vi "ControlPanel.vi"(0 "NXT":T1={"Hardware"="NXT", "Flattened String"=""}) -> (5 "NXT":T1={"Hardware"="NXT", "Flattened String"=""})   [LabVIEW 2010]
uses:
  <vilib>/NXT/Block Support/NXT_InputPort.ctl
  <vilib>/NXT/Subs/LVHSConnector.ctl
  <vilib>/NXT/Block Support/NXT_ButtonSelector.ctl
  <vilib>/NXT/Subs/MotorXNode.DC Motor Type.ctl
  <vilib>/NXT/NXTIO Xnodes/NXTIOXNode/NXTIO.xnode
  <vilib>/NXT/Subs/MotorXNode.1DCMotor.ctl
  <vilib>/NXT/Subs/MotorXNode.Servo Type.ctl
  <vilib>/NXT/Subs/MotorXNode.1Servo.ctl
  <vilib>/NXT/Dual Mode Library/Waits/Wait_Num(msec).vi
  <vilib>/NXT/Dual Mode Library/Display/clearDisplay.vi
  <vilib>/NXT/Dual Mode Library/Waits/Wait_Btn_Release.vi
  <vilib>/NXT/Dual Mode Library/Display/drawText.vi
  <vilib>/NXT/Dual Mode Library/Display/drawNumber.vi
  <vilib>/NXT/Dual Mode Library/Display/drawNumber_float.vi
  <vilib>/NXT/NXTIO Xnodes/NXTIONodeSubVIs/TETRIX IO Move DC Motors.vi
  <vilib>/NXT/NXTIO Xnodes/NXTIONodeSubVIs/TETRIX IO Motor Status.vi
  <vilib>/NXT/NXTIO Xnodes/NXTIONodeSubVIs/TETRIX IO Move Servos.vi
  Components/Components.lvlib
panel:
  out "exit?":bool
  out "Enter":bool caption="Yes/No"
  out "Right":bool caption="Yes/No"
  out "Left":bool caption="Yes/No"
  in  "Sensor Type":T2(ring)
  in  "MUX Port":u8(ring) items=["No MUX", "MUX 1", "MUX 2", "MUX 3", "MUX 4"]
  in  "Sensor Port":T3 items=["Port 1", "Port 2", "Port 3", "Port 4"]
  in  "Motor Port":u8(ring)=1 items=["A", "B", "C"]
  in  "Type":T4(ring)
  in  "Controller Slot":u8(ring)=1 items=["1"=1, "2"=2, "3"=3, "4"=4, "5"=5, "6"=6]
  in  "Chain Position":u8(ring)=1 items=["1"=1, "2"=2, "3"=3, "4"=4]
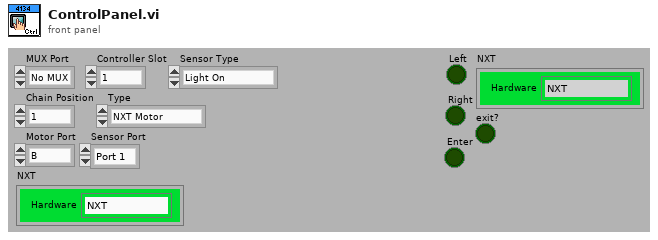
[diagram p1: front panel]
types:
  T1 = typedef "LVHSConnector.ctl" = cluster{"Hardware":string, "Flattened String":string}
  T2 = enum16{"Light On", "Light Off", "Touch", "Sound", "Ultrasonic", "Accelerometer", "Compass", "EOPD", "Force", "Gyro", "IR v1", "IR v2"}
  T3 = typedef "NXT_InputPort.ctl" = u8
  T4 = enum16{"NXT Motor", "NXT Rotation Sensor", "NXT Sensor", "NXT Battery", "Tetrix Motor", "Tetrix Servo", "Tetrix Encoder", "Tetrix Battery"}
  T5 = typedef "MotorXNode.DC Motor Type.ctl" = enum16{"DC Motor"}
  T6 = typedef "MotorXNode.Servo Type.ctl" = enum16{"Servo"}
  T7 = cluster{"Direction (0-9)":i16, "Signal Strength (Array)":u8[]}
  T8 = typedef "NXT_ButtonSelector.ctl" = u16
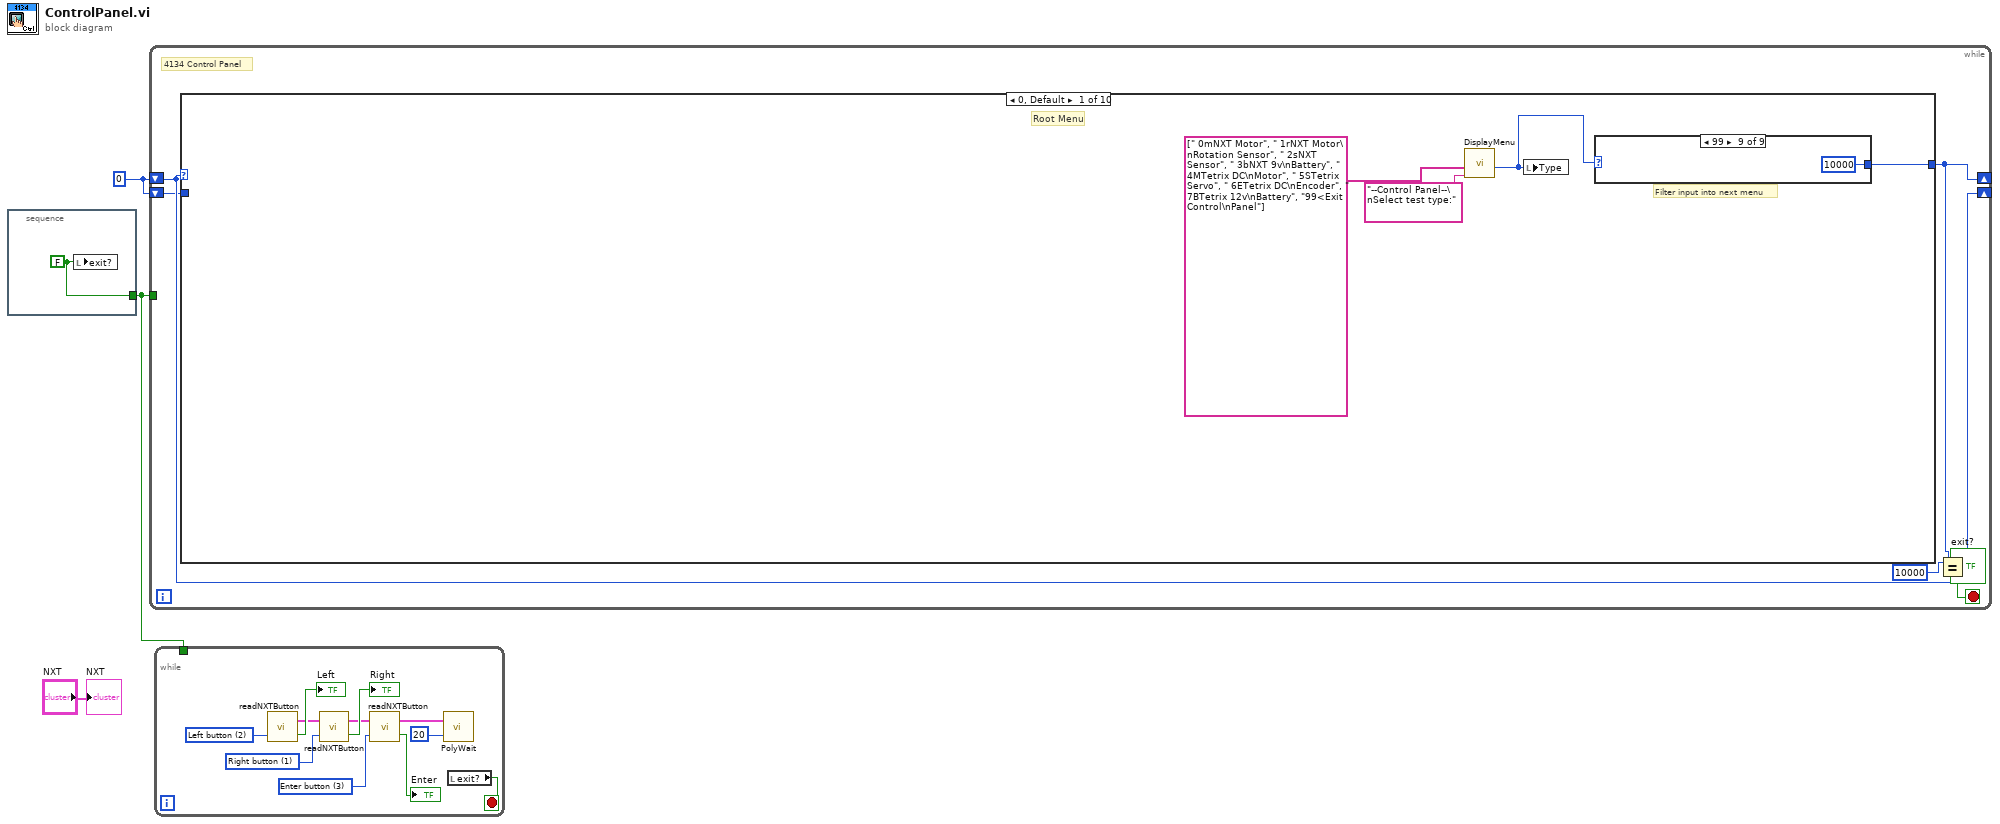
[diagram p0: block diagram]
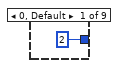
[diagram p2: hidden frame]
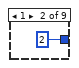
[diagram p3: hidden frame]
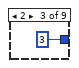
[diagram p4: hidden frame]
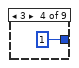
[diagram p5: hidden frame]
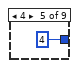
[diagram p6: hidden frame]
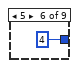
[diagram p7: hidden frame]
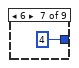
[diagram p8: hidden frame]
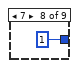
[diagram p9: hidden frame]
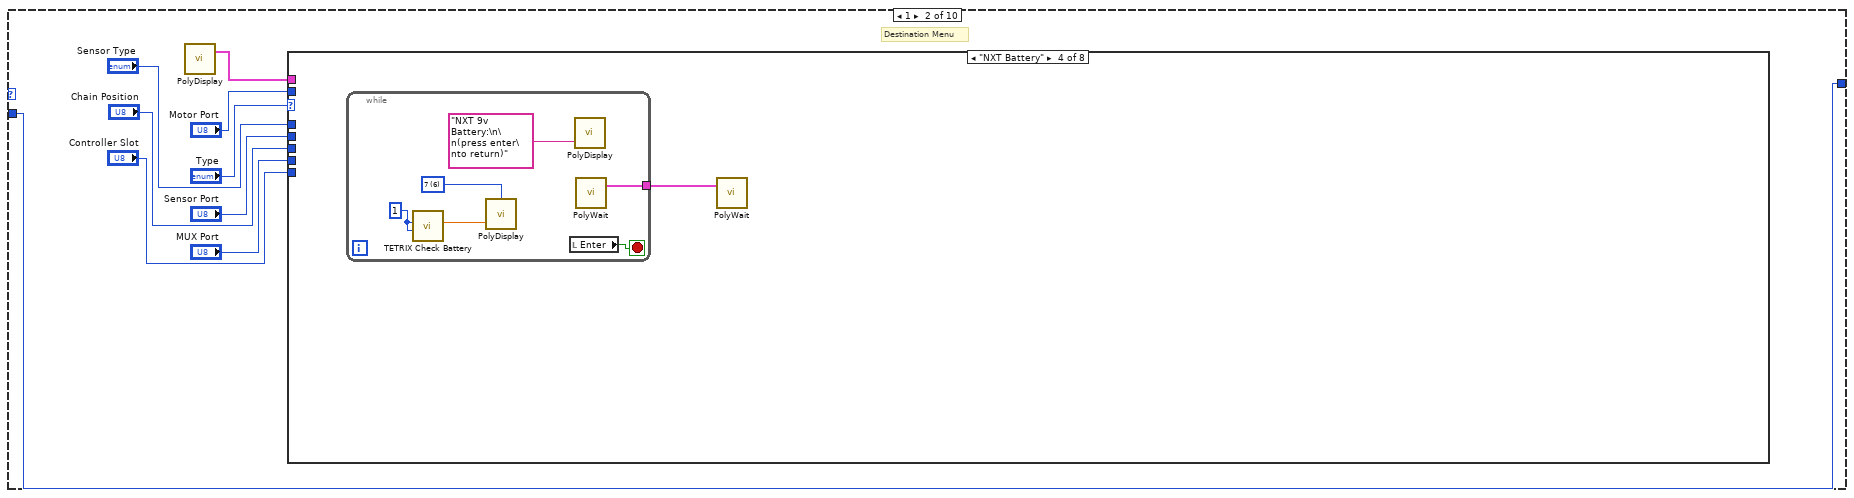
[diagram p10: hidden frame]
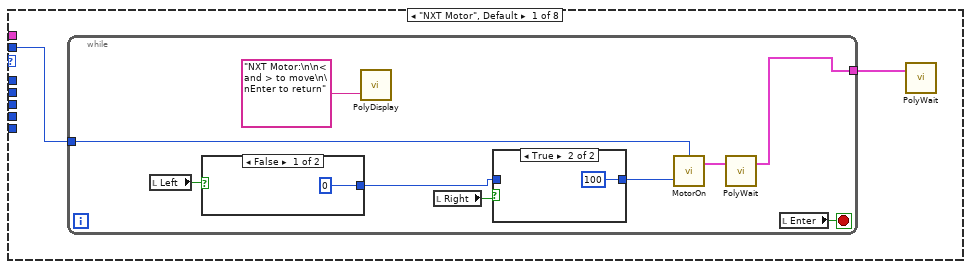
[diagram p11: hidden frame]
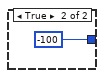
[diagram p13: hidden frame]
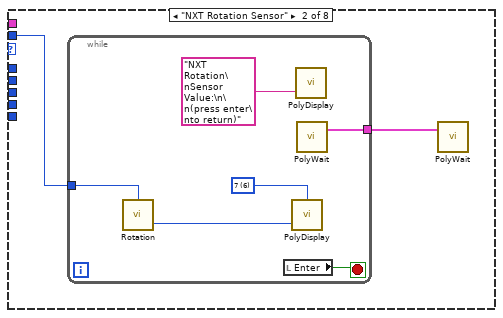
[diagram p14: hidden frame]
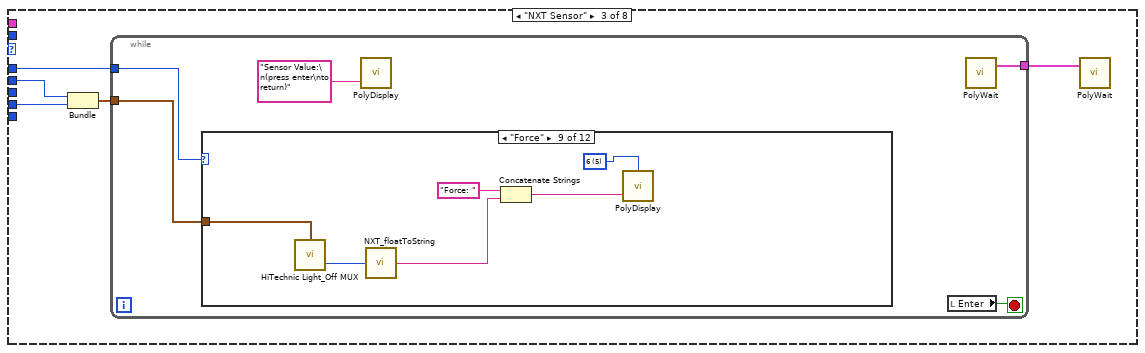
[diagram p15: hidden frame]
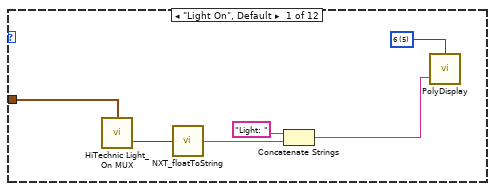
[diagram p16: hidden frame]
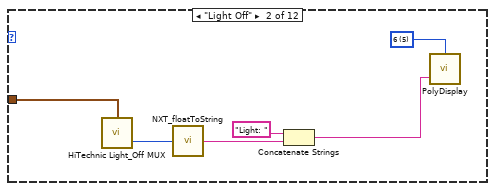
[diagram p17: hidden frame]
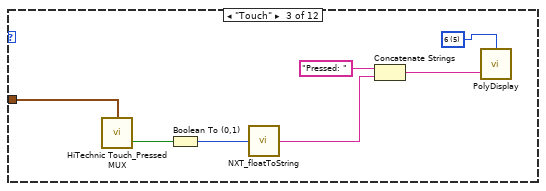
[diagram p18: hidden frame]
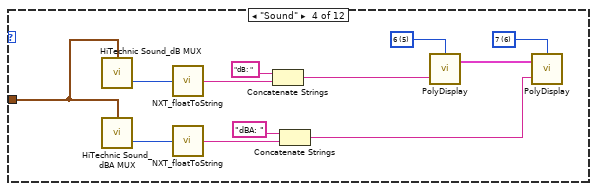
[diagram p19: hidden frame]
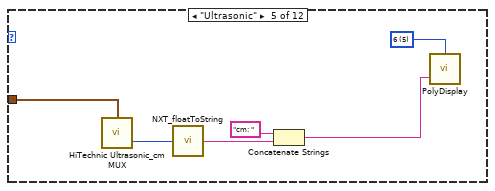
[diagram p20: hidden frame]
diagram:
  w3 = u32 0 ("Selected ID")
  n1 = stacked-sequence {
    tunnel: [w4] -> w1
    frame #0 {
      w4 = FALSE ("exit?")
      n2 = local write "exit?"(w4) -> ()
    }
  }
  n3 = while {
    shift-right: [w7] -> _
    shift-left: w3 -> [w9]
    shift-right: [w9] -> _
    shift-left: w3 -> [w8]
    tunnel: w1 -> [_]
    stop <- w6 stop-if-true
    # "4134 Control Panel"
    n4 = case shown="0, Default" w9 {
      tunnel: [w11 w30 w336 w343 w350 w357 w366 w375 w382 w389] -> w7
      tunnel: w8 -> [_ w30 _ _ _ _ _ _ _ _]
      frame 0, Default {
        # "Filter input into next menu"
        # "Root Menu"
        n5 = call "DisplayMenu.vi"("Menu Message"="--Control Panel--\nSelect test type:", "2-Digit ID+Character+Message"=string[] [" 0mNXT Motor", " 1rNXT Motor\nRotation Sensor", " 2sNXT Sensor", " 3bNXT 9v\nBattery", " 4MTetrix DC\nMotor", " 5STetrix Servo", " 6ETetrix DC\nEncoder", " 7BTetrix 12v\nBattery", "99<Exit Control\nPanel"] ("Array")) -> ("Selected ID"=w12:i32)  [unwired: 6 in, 1 out]
        n6 = local write "Type"(w12) -> ()
        n7 = case shown="99" w12 {
          tunnel: [2 2 3 1 4 4 4 1 10000] -> w11
          frame 0, Default {
          }
          frame 1 {
          }
          frame 2 {
          }
          frame 3 {
          }
          frame 4 {
          }
          frame 5 {
          }
          frame 6 {
          }
          frame 7 {
          }
          frame 99 {
          }
        }
      }
      frame 1 {
        # "Destination Menu"
        n8 = call-poly <vilib>:"PolyDisplay.vi"() -> ("NXT"=w29:T1)  [unwired: 4 in]
        n9 = case shown="\"NXT Battery\"" "Type" {
          tunnel: w29 -> [_ _ _ _ _ _ _ _]
          tunnel: "Motor Port" -> [w32 w47 _ _ _ _ _ _]
          tunnel: "Sensor Port" -> [_ _ w57 _ w188 w223 w269 _]
          tunnel: "MUX Port" -> [_ _ w58 _ _ _ _ _]
          tunnel: "Chain Position" -> [_ _ _ _ w185 w220 w266 _]
          tunnel: "Controller Slot" -> [_ _ _ _ w184 w219 w265 _]
          tunnel: "Sensor Type" -> [_ _ w59 _ _ _ _ _]
          frame "NXT Motor", Default {
            n10 = while {
              tunnel: [w41] -> w33
              tunnel: w32 -> [w38]
              stop <- w34 stop-if-true
              n11 = local read "Left"() -> (w36:bool)
              n12 = case shown="False" w36 {
                tunnel: [0 -100] -> w40
                frame False {
                }
                frame True {
                }
              }
              n13 = call-poly <vilib>:"PolyDisplay.vi"("Text"="NXT Motor:\n\n< and > to move\n\nEnter to return") -> ()  [unwired: 3 in, 1 out]
              n14 = local read "Right"() -> (w35:bool)
              n15 = case shown="True" w35 {
                tunnel: w40 -> [w43 _]
                tunnel: [w43 100] -> w39
                frame False {
                }
                frame True {
                }
              }
              n16 = call <vilib>:"MotorOn.vi"("Power (75)"=w39, "Output Port (All Ports)"=w38) -> ("NXT"=w37:T1)  [unwired: 2 in]
              n17 = call-poly <vilib>:"PolyWait.vi"("NXT"=w37) -> ("NXT"=w41:T1)  [unwired: 3 in]
              n18 = local read "Enter"() -> (w34:bool)
            }
            n19 = call-poly <vilib>:"PolyWait.vi"("NXT"=w33) -> ()  [unwired: 3 in, 1 out]
          }
          frame "NXT Rotation Sensor" {
            n20 = while {
              tunnel: [w52] -> w48
              tunnel: w47 -> [w50]
              stop <- w49 stop-if-true
              w54 = i16 6 items=["1", "2", "3", "4", "5", "6", "7", "8"] ("Line")
              n21 = call <vilib>:"Rotation.vi"("Port (Port A)"=w50) -> ("Angle of Rotation"=w51:i32)  [unwired: 2 in, 1 out]
              n22 = local read "Enter"() -> (w49:bool)
              n23 = call-poly <vilib>:"PolyDisplay.vi"("number"=w51, "Line"=w54) -> ()  [unwired: 2 in, 1 out]
              n24 = call-poly <vilib>:"PolyDisplay.vi"("Text"="NXT Rotation\nSensor Value:\n\n(press enter\nto return)") -> ()  [unwired: 3 in, 1 out]
              n25 = call-poly <vilib>:"PolyWait.vi"() -> ("NXT"=w52:T1)  [unwired: 4 in]
            }
            n26 = call-poly <vilib>:"PolyWait.vi"("NXT"=w48) -> ()  [unwired: 3 in, 1 out]
          }
          frame "NXT Sensor" {
            n27 = Bundle("Sensor Port"=w57, "MUX Port"=w58) -> (w56:cluster{"Sensor Port":T3, "MUX Port":u8})  [unwired: 1 in]
            n28 = while {
              tunnel: w59 -> [w62]
              tunnel: w56 -> [w61]
              tunnel: [w64] -> w55
              stop <- w60 stop-if-true
              n29 = case shown="\"Force\"" w62 {
                tunnel: w61 -> [w70 w71 w79 w90 w96 w118 w120 w129 w138 w144 w152 w161]
                frame "Light On", Default {
                  w65 = i16 5 items=["1", "2", "3", "4", "5", "6", "7", "8"] ("Line")
                  n30 = call <vilib>:"HiTechnic Light_On MUX.vi"("Port/MUX"=w70) -> ("Scaled Value"=w69:i16)  [unwired: 2 in, 1 out]
                  n31 = call <vilib>:"NXT_floatToString.vi"("number"=w69) -> ("string"=w68:string)
                  n32 = Concatenate Strings("Light: ", w68) -> (w66:string)
                  n33 = call-poly <vilib>:"PolyDisplay.vi"("Text"=w66, "Line"=w65) -> ()  [unwired: 2 in, 1 out]
                }
                frame "Light Off" {
                  w72 = i16 5 items=["1", "2", "3", "4", "5", "6", "7", "8"] ("Line")
                  n34 = call <vilib>:"HiTechnic Light_Off MUX.vi"("Port/MUX"=w71) -> ("Scaled Value"=w76:i16)  [unwired: 2 in, 1 out]
                  n35 = call <vilib>:"NXT_floatToString.vi"("number"=w76) -> ("string"=w75:string)
                  n36 = Concatenate Strings("Light: ", w75) -> (w73:string)
                  n37 = call-poly <vilib>:"PolyDisplay.vi"("Text"=w73, "Line"=w72) -> ()  [unwired: 2 in, 1 out]
                }
                frame "Touch" {
                  w80 = i16 5 items=["1", "2", "3", "4", "5", "6", "7", "8"] ("Line")
                  n38 = call <vilib>:"HiTechnic Touch_Pressed MUX.vi"("Port/MUX"=w79) -> ("Yes / No"=w78:bool)  [unwired: 2 in, 1 out]
                  n39 = Boolean To (0,1)(Boolean=w78) -> (0, 1=w77:i16)
                  n40 = call <vilib>:"NXT_floatToString.vi"("number"=w77) -> ("string"=w83:string)
                  n41 = Concatenate Strings("Pressed: ", w83) -> (w81:string)
                  n42 = call-poly <vilib>:"PolyDisplay.vi"("Text"=w81, "Line"=w80) -> ()  [unwired: 2 in, 1 out]
                }
                frame "Sound" {
                  w84 = i16 6 items=["1", "2", "3", "4", "5", "6", "7", "8"] ("Line")
                  w91 = i16 5 items=["1", "2", "3", "4", "5", "6", "7", "8"] ("Line")
                  n43 = call <vilib>:"HiTechnic Sound_dB MUX.vi"("Port/MUX"=w90) -> ("Scaled Value"=w95:i16)  [unwired: 2 in, 1 out]
                  n44 = call <vilib>:"HiTechnic Sound_dBA MUX.vi"("Port/MUX"=w90) -> ("Scaled Value"=w89:i16)  [unwired: 2 in, 1 out]
                  n45 = call <vilib>:"NXT_floatToString.vi"("number"=w95) -> ("string"=w94:string)
                  n46 = call <vilib>:"NXT_floatToString.vi"("number"=w89) -> ("string"=w88:string)
                  n47 = Concatenate Strings("dB: ", w94) -> (w92:string)
                  n48 = Concatenate Strings("dBA: ", w88) -> (w85:string)
                  n49 = call-poly <vilib>:"PolyDisplay.vi"("Text"=w92, "Line"=w91) -> ("NXT"=w86:T1)  [unwired: 2 in]
                  n50 = call-poly <vilib>:"PolyDisplay.vi"("Text"=w85, "NXT"=w86, "Line"=w84) -> ()  [unwired: 1 in, 1 out]
                }
                frame "Ultrasonic" {
                  w97 = i16 5 items=["1", "2", "3", "4", "5", "6", "7", "8"] ("Line")
                  n51 = call <vilib>:"HiTechnic Ultrasonic_cm MUX.vi"("Port/MUX"=w96) -> ("Distance (cm)"=w101:i16)  [unwired: 2 in, 1 out]
                  n52 = call <vilib>:"NXT_floatToString.vi"("number"=w101) -> ("string"=w100:string)
                  n53 = Concatenate Strings("cm: ", w100) -> (w98:string)
                  n54 = call-poly <vilib>:"PolyDisplay.vi"("Text"=w98, "Line"=w97) -> ()  [unwired: 2 in, 1 out]
                }
                frame "Accelerometer" {
                  w114 = i16 7 items=["1", "2", "3", "4", "5", "6", "7", "8"] ("Line")
                  w115 = i16 6 items=["1", "2", "3", "4", "5", "6", "7", "8"] ("Line")
                  w119 = i16 5 items=["1", "2", "3", "4", "5", "6", "7", "8"] ("Line")
                  n55 = call <vilib>:"HiTechnic Acceleration Sensor.vi"("Port/MUX"=w118) -> ("Z Acceleration (m/s^2)"=w102:sgl, "Y Acceleration (m/s^2)"=w105:sgl, "X Acceleration (m/s^2)"=w107:sgl)  [unwired: 3 in, 1 out]
                  n56 = call <vilib>:"NXT_floatToString.vi"("number"=w107) -> ("string"=w106:string)
                  n57 = call <vilib>:"NXT_floatToString.vi"("number"=w105) -> ("string"=w104:string)
                  n58 = call <vilib>:"NXT_floatToString.vi"("number"=w102) -> ("string"=w103:string)
                  n59 = Concatenate Strings("X: ", w106) -> (w111:string)
                  n60 = Concatenate Strings("Y: ", w104) -> (w113:string)
                  n61 = Concatenate Strings("Z: ", w103) -> (w112:string)
                  n62 = call-poly <vilib>:"PolyDisplay.vi"("Text"=w111, "Line"=w119) -> ("NXT"=w117:T1)  [unwired: 2 in]
                  n63 = call-poly <vilib>:"PolyDisplay.vi"("Text"=w113, "NXT"=w117, "Line"=w115) -> ("NXT"=w116:T1)  [unwired: 1 in]
                  n64 = call-poly <vilib>:"PolyDisplay.vi"("Text"=w112, "NXT"=w116, "Line"=w114) -> ()  [unwired: 1 in, 1 out]
                }
                frame "Compass" {
                  w121 = i16 5 items=["1", "2", "3", "4", "5", "6", "7", "8"] ("Line")
                  n65 = call <vilib>:"HiTechnic Compass Sensor.vi"("Port/MUX"=w120) -> ("Heading (degrees)"=w125:i16)  [unwired: 2 in, 1 out]
                  n66 = call <vilib>:"NXT_floatToString.vi"("number"=w125) -> ("string"=w124:string)
                  n67 = Concatenate Strings("Deg: ", w124) -> (w122:string)
                  n68 = call-poly <vilib>:"PolyDisplay.vi"("Text"=w122, "Line"=w121) -> ()  [unwired: 2 in, 1 out]
                }
                frame "EOPD" {
                  w126 = i16 6 items=["1", "2", "3", "4", "5", "6", "7", "8"] ("Line")
                  w133 = i16 5 items=["1", "2", "3", "4", "5", "6", "7", "8"] ("Line")
                  n69 = call <vilib>:"HiTechnic EOPD Sensor Long.vi"("Port/MUX"=w129) -> ("EOPD Value"=w137:i16)  [unwired: 2 in, 1 out]
                  n70 = call <vilib>:"HiTechnic EOPD Sensor Short.vi"("Port/MUX"=w129) -> ("EOPD Value"=w130:i16)  [unwired: 2 in, 1 out]
                  n71 = call <vilib>:"NXT_floatToString.vi"("number"=w137) -> ("string"=w136:string)
                  n72 = call <vilib>:"NXT_floatToString.vi"("number"=w130) -> ("string"=w131:string)
                  n73 = Concatenate Strings("Long: ", w136) -> (w134:string)
                  n74 = Concatenate Strings("Short: ", w131) -> (w128:string)
                  n75 = call-poly <vilib>:"PolyDisplay.vi"("Text"=w134, "Line"=w133) -> ("NXT"=w127:T1)  [unwired: 2 in]
                  n76 = call-poly <vilib>:"PolyDisplay.vi"("Text"=w128, "NXT"=w127, "Line"=w126) -> ()  [unwired: 1 in, 1 out]
                }
                frame "Force" {
                  w139 = i16 5 items=["1", "2", "3", "4", "5", "6", "7", "8"] ("Line")
                  n77 = call <vilib>:"HiTechnic Light_Off MUX.vi"("Port/MUX"=w138) -> ("Scaled Value"=w143:i16)  [unwired: 2 in, 1 out]
                  n78 = call <vilib>:"NXT_floatToString.vi"("number"=w143) -> ("string"=w142:string)
                  n79 = Concatenate Strings("Force: ", w142) -> (w140:string)
                  n80 = call-poly <vilib>:"PolyDisplay.vi"("Text"=w140, "Line"=w139) -> ()  [unwired: 2 in, 1 out]
                }
                frame "Gyro" {
                  w145 = i16 5 items=["1", "2", "3", "4", "5", "6", "7", "8"] ("Line")
                  n81 = call <vilib>:"HiTechnic Gyro Sensor.vi"("Port/MUX"=w144) -> ("Gyro Value"=w149:i16)  [unwired: 2 in, 1 out]
                  n82 = call <vilib>:"NXT_floatToString.vi"("number"=w149) -> ("string"=w148:string)
                  n83 = Concatenate Strings("Deg/s: ", w148) -> (w146:string)
                  n84 = call-poly <vilib>:"PolyDisplay.vi"("Text"=w146, "Line"=w145) -> ()  [unwired: 2 in, 1 out]
                }
                frame "IR v1" {
                  w153 = i16 5 items=["1", "2", "3", "4", "5", "6", "7", "8"] ("Line")
                  n85 = call <vilib>:"HiTechnic IRSeeker Sensor_V1 all.vi"("Port/MUX"=w152) -> ("All Info"=w151:T7)  [unwired: 2 in, 1 out]
                  n86 = Unbundle(w151) -> ("Direction (0-9)"=w150:i16)  [unwired: 1 out]
                  n87 = call <vilib>:"NXT_floatToString.vi"("number"=w150) -> ("string"=w156:string)
                  n88 = Concatenate Strings("Seg: ", w156) -> (w154:string)
                  n89 = call-poly <vilib>:"PolyDisplay.vi"("Text"=w154, "Line"=w153) -> ()  [unwired: 2 in, 1 out]
                }
                frame "IR v2" {
                  w162 = i16 6 items=["1", "2", "3", "4", "5", "6", "7", "8"] ("Line")
                  w167 = i16 5 items=["1", "2", "3", "4", "5", "6", "7", "8"] ("Line")
                  n90 = call <vilib>:"HiTechnic IRSeeker Sensor_AC all.vi"("Port/MUX"=w161) -> ("All Info"=w160:T7)  [unwired: 2 in, 1 out]
                  n91 = call <vilib>:"HiTechnic IRSeeker Sensor_DC all.vi"("Port/MUX"=w161) -> ("All Info"=w158:T7)  [unwired: 2 in, 1 out]
                  n92 = Unbundle(w160) -> ("Direction (0-9)"=w159:i16)  [unwired: 1 out]
                  n93 = Unbundle(w158) -> ("Direction (0-9)"=w157:i16)  [unwired: 1 out]
                  n94 = call <vilib>:"NXT_floatToString.vi"("number"=w159) -> ("string"=w170:string)
                  n95 = call <vilib>:"NXT_floatToString.vi"("number"=w157) -> ("string"=w165:string)
                  n96 = Concatenate Strings("AC: ", w170) -> (w168:string)
                  n97 = Concatenate Strings("DC: ", w165) -> (w164:string)
                  n98 = call-poly <vilib>:"PolyDisplay.vi"("Text"=w168, "Line"=w167) -> ("NXT"=w163:T1)  [unwired: 2 in]
                  n99 = call-poly <vilib>:"PolyDisplay.vi"("Text"=w164, "NXT"=w163, "Line"=w162) -> ()  [unwired: 1 in, 1 out]
                }
              }
              n100 = call-poly <vilib>:"PolyDisplay.vi"("Text"="Sensor Value:\n(press enter\nto return)") -> ()  [unwired: 3 in, 1 out]
              n101 = local read "Enter"() -> (w60:bool)
              n102 = call-poly <vilib>:"PolyWait.vi"() -> ("NXT"=w64:T1)  [unwired: 4 in]
            }
            n103 = call-poly <vilib>:"PolyWait.vi"("NXT"=w55) -> ()  [unwired: 3 in, 1 out]
          }
          frame "NXT Battery" {
            n104 = while {
              tunnel: [w175] -> w171
              stop <- w172 stop-if-true
              w174 = u8 1 ("Motor Controller")
              w177 = i16 6 items=["1", "2", "3", "4", "5", "6", "7", "8"] ("Line")
              n105 = call <vilib>:"TETRIX Check Battery.vi"("Motor Controller"=w174, "Port"=w174) -> ("NXT Voltage"=w173:dbl)  [unwired: 7 in, 2 out]
              n106 = call-poly <vilib>:"PolyDisplay.vi"("number"=w173, "Line"=w177) -> ()  [unwired: 2 in, 1 out]
              n107 = local read "Enter"() -> (w172:bool)
              n108 = call-poly <vilib>:"PolyDisplay.vi"("Text"="NXT 9v Battery:\n\n(press enter\nto return)") -> ()  [unwired: 3 in, 1 out]
              n109 = call-poly <vilib>:"PolyWait.vi"() -> ("NXT"=w175:T1)  [unwired: 4 in]
            }
            n110 = call-poly <vilib>:"PolyWait.vi"("NXT"=w171) -> ()  [unwired: 3 in, 1 out]
          }
          frame "Tetrix Motor" {
            n111 = Multiply(x=w188, y=i16 1000) -> (x*y=w183:i16)
            n112 = Multiply(x=w185, y=i16 100) -> (x*y=w182:i16)
            n113 = Add(x=w183, y=w182) -> (x+y=w181:i16)
            n114 = Multiply(x=w184, y=i16 10) -> (x*y=w180:i16)
            n115 = Add(x=w181, y=w180) -> (x+y=w178:i16)
            n116 = while {
              tunnel: [w199] -> w179
              tunnel: w178 -> [w193]
              stop <- w192 stop-if-true
              n117 = local read "Left"() -> (w191:bool)
              n118 = case shown="False" w191 {
                tunnel: [0 -100] -> w198
                frame False {
                }
                frame True {
                }
              }
              n119 = call-poly <vilib>:"PolyDisplay.vi"("Text"="Tetrix Motor:\n\n< and > to move\n\nEnter to return") -> ()  [unwired: 3 in, 1 out]
              n120 = local read "Right"() -> (w190:bool)
              n121 = case shown="True" w190 {
                tunnel: w198 -> [w209 _]
                tunnel: [w209 100] -> w197
                frame False {
                }
                frame True {
                }
              }
              n122 = Bundle(cluster=cluster{"DC Motor":T5, "Address":i16} {"DC Motor"=enum."DC Motor", "Address"=-1} ("DC Motor"), "Address"=w193) -> (w194:cluster{"DC Motor":T5, "Address":i16})  [unwired: 1 in]
              n123 = xnode "Move DC Motors"("Power/Speed 1"=w197, "Motors"=w194) -> ("NXT"=w196:T1)  [unwired: 1 in]
              n124 = call-poly <vilib>:"PolyWait.vi"("NXT"=w196) -> ("NXT"=w199:T1)  [unwired: 3 in]
              n125 = local read "Enter"() -> (w192:bool)
            }
            n126 = call-poly <vilib>:"PolyWait.vi"("NXT"=w179) -> ()  [unwired: 3 in, 1 out]
          }
          frame "Tetrix Encoder" {
            n127 = Multiply(x=w223, y=i16 1000) -> (x*y=w218:i16)
            n128 = Multiply(x=w220, y=i16 100) -> (x*y=w217:i16)
            n129 = Add(x=w218, y=w217) -> (x+y=w216:i16)
            n130 = Multiply(x=w219, y=i16 10) -> (x*y=w215:i16)
            n131 = Add(x=w216, y=w215) -> (x+y=w213:i16)
            n132 = while {
              tunnel: [w235] -> w214
              tunnel: w213 -> [w230]
              stop <- w225 stop-if-true
              w233 = i16 7 items=["1", "2", "3", "4", "5", "6", "7", "8"] ("Line")
              n133 = Bundle(cluster=cluster{"DC Motor":T5, "Address":i16} {"DC Motor"=enum."DC Motor", "Address"=-1} ("DC Motor"), "Address"=w230) -> (w228:cluster{"DC Motor":T5, "Address":i16})  [unwired: 1 in]
              n134 = xnode "Motor Status"("Motors"=w228) -> ("Position 1"=w232:i32)  [unwired: 1 in, 2 out]
              n135 = local read "Left"() -> (w227:bool)
              n136 = case shown="False" w227 {
                tunnel: [0 -100] -> w234
                frame False {
                }
                frame True {
                }
              }
              n137 = call-poly <vilib>:"PolyDisplay.vi"("number"=w232, "Line"=w233) -> ()  [unwired: 2 in, 1 out]
              n138 = call-poly <vilib>:"PolyDisplay.vi"("Text"="Tetrix Encoder:\n\n< and > to move\n\nEnter to return") -> ()  [unwired: 3 in, 1 out]
              n139 = local read "Right"() -> (w226:bool)
              n140 = case shown="True" w226 {
                tunnel: w234 -> [w254 _]
                tunnel: [w254 100] -> w229
                frame False {
                }
                frame True {
                }
              }
              n141 = xnode "Move DC Motors"("Power/Speed 1"=w229, "Motors"=w228) -> ()  [unwired: 1 in, 1 out]
              n142 = local read "Enter"() -> (w225:bool)
              n143 = call-poly <vilib>:"PolyWait.vi"() -> ("NXT"=w235:T1)  [unwired: 4 in]
            }
            n144 = call-poly <vilib>:"PolyWait.vi"("NXT"=w214) -> ()  [unwired: 3 in, 1 out]
          }
          frame "Tetrix Servo" {
            n145 = Multiply(x=w269, y=i16 1000) -> (x*y=w264:i16)
            n146 = Multiply(x=w266, y=i16 100) -> (x*y=w263:i16)
            n147 = Add(x=w264, y=w263) -> (x+y=w262:i16)
            n148 = Multiply(x=w265, y=i16 10) -> (x*y=w261:i16)
            n149 = Add(x=w262, y=w261) -> (x+y=w258:i16)
            n150 = while {
              tunnel: [w288] -> w260
              tunnel: w258 -> [w276]
              shift-right: [w274] -> _
              shift-left: 0 -> [w279]
              stop <- w271 stop-if-true
              w287 = i16 7 items=["1", "2", "3", "4", "5", "6", "7", "8"] ("Line")
              n151 = Greater Than 0?(x=w279) -> (x > 0?=w281:bool)
              n152 = local read "Right"() -> (w273:bool)
              n153 = Less?(x=w279, y=255) -> (x < y?=w284:bool)
              n154 = local read "Left"() -> (w272:bool)
              n155 = And(x=w284, y=w273) -> (x .and. y?=w283:bool)
              n156 = And(x=w281, y=w272) -> (x .and. y?=w282:bool)
              n157 = case shown="True" w282 {
                tunnel: w279 -> [w301 w302]
                tunnel: [w301 w303] -> w280
                frame False {
                }
                frame True {
                  n158 = Decrement(x=w302) -> (x-1=w303:i32)
                }
              }
              n159 = call-poly <vilib>:"PolyDisplay.vi"("Text"="Tetrix Servo:\n\n< and > to move\n\nEnter to return") -> ()  [unwired: 3 in, 1 out]
              n160 = case shown="True" w283 {
                tunnel: [w298 w300] -> w274
                tunnel: w280 -> [w298 w299]
                frame False {
                }
                frame True {
                  n161 = Increment(x=w299) -> (x+1=w300:i32)
                }
              }
              n162 = Bundle(cluster=cluster{"Servo":T6, "Address":i16} {"Servo"=enum."Servo", "Address"=-1} ("Servo"), "Address"=w276) -> (w275:cluster{"Servo":T6, "Address":i16})  [unwired: 1 in]
              n163 = call-poly <vilib>:"PolyDisplay.vi"("number"=w274, "Line"=w287) -> ()  [unwired: 2 in, 1 out]
              n164 = xnode "Move Servos"("Position 1"=w274, "Servos"=w275) -> ("NXT"=w278:T1)  [unwired: 1 in]
              n165 = call-poly <vilib>:"PolyWait.vi"("Time (100 msec)"=u32 10, "NXT"=w278) -> ("NXT"=w288:T1)  [unwired: 2 in]
              n166 = local read "Enter"() -> (w271:bool)
            }
            n167 = call-poly <vilib>:"PolyWait.vi"("NXT"=w260) -> ()  [unwired: 3 in, 1 out]
          }
          frame "Tetrix Battery" {
            n168 = while {
              shift-right: [w311] -> _
              shift-left: 0 -> [w313]
              tunnel: [w324] -> w304
              stop <- w308 stop-if-true
              w319 = i16 5 items=["1", "2", "3", "4", "5", "6", "7", "8"] ("Line")
              w327 = i16 7 items=["1", "2", "3", "4", "5", "6", "7", "8"] ("Line")
              n169 = Greater Than 0?(x=w313) -> (x > 0?=w317:bool)
              n170 = Increment(x=w313) -> (x+1=w323:i32)
              n171 = Less?(x=w313, y=3) -> (x < y?=w314:bool)
              n172 = call <vilib>:"TETRIX Check Battery.vi"("Motor Controller"=u8 1, "Port"=w313) -> ("Motor Controller Voltage"=w328:dbl)  [unwired: 7 in, 2 out]
              n173 = local read "Left"() -> (w307:bool)
              n174 = local read "Right"() -> (w306:bool)
              n175 = call <vilib>:"NXT_floatToString.vi"("number"=w323) -> ("string"=w322:string)
              n176 = call-poly <vilib>:"PolyDisplay.vi"("Text"="Tetrix 12v\nBattery:\n(press enter\nto return)") -> ()  [unwired: 3 in, 1 out]
              n177 = And(x=w317, y=w307) -> (x .and. y?=w316:bool)
              n178 = And(x=w314, y=w306) -> (x .and. y?=w315:bool)
              n179 = call-poly <vilib>:"PolyDisplay.vi"("number"=w328, "Line"=w327) -> ()  [unwired: 2 in, 1 out]
              n180 = case shown="True" w316 {
                tunnel: w313 -> [w332 w333]
                tunnel: [w332 w334] -> w312
                frame False {
                }
                frame True {
                  n181 = Decrement(x=w333) -> (x-1=w334:i32)
                }
              }
              n182 = Concatenate Strings("<  Port ", w322, "  >") -> (w320:string)
              n183 = case shown="False" w315 {
                tunnel: [w329 w331] -> w311
                tunnel: w312 -> [w329 w330]
                frame False {
                }
                frame True {
                  n184 = Increment(x=w330) -> (x+1=w331:i32)
                }
              }
              n185 = call-poly <vilib>:"PolyDisplay.vi"("Text"=w320, "Line"=w319) -> ()  [unwired: 2 in, 1 out]
              n186 = call-poly <vilib>:"PolyWait.vi"("Time (100 msec)"=u32 200) -> ("NXT"=w324:T1)  [unwired: 3 in]
              n187 = local read "Enter"() -> (w308:bool)
            }
            n188 = call-poly <vilib>:"PolyWait.vi"("NXT"=w304) -> ()  [unwired: 3 in, 1 out]
          }
        }
      }
      frame 2 {
        # "NXT Motor or Rotation Sensor"
        n189 = call "DisplayMenu.vi"("Menu Message"="--Select Port--", "2-Digit ID+Character+Message"=string[] [" 0AMotor Port A", " 1BMotor Port B", " 2CMotor Port C", "10<Return"] ("Array")) -> ("Selected ID"=w337:i32)  [unwired: 6 in, 1 out]
        n190 = case shown="10" w337 {
          selector: w337 -> [w340 _]
          tunnel: [u32 1 ("Selected ID") 0] -> w336
          frame 0, Default {
            n191 = local write "Motor Port"(w340) -> ()
          }
          frame 10 {
          }
        }
      }
      frame 3 {
        # "NXT Sensor (besides rotation) - root"
        n192 = call "DisplayMenu.vi"("Menu Message"="--Select Port--", "2-Digit ID+Character+Message"=string[] [" 01Sensor Port 1", " 12Sensor Port 2", " 23Sensor Port 3", " 34Sensor Port 4", "10<Return"] ("Array")) -> ("Selected ID"=w344:i32)  [unwired: 6 in, 1 out]
        n193 = case shown="0, Default" w344 {
          selector: w344 -> [w347 _]
          tunnel: [u32 5 ("Selected ID") 0] -> w343
          frame 0, Default {
            n194 = local write "Sensor Port"(w347) -> ()
          }
          frame 10 {
          }
        }
      }
      frame 4 {
        # "Tetrix Motor, Servo, or Encoder - port"
        n195 = call "DisplayMenu.vi"("Menu Message"="--Select Port--", "2-Digit ID+Character+Message"=string[] [" 11Sensor Port 1", " 22Sensor Port 2", " 33Sensor Port 3", " 44Sensor Port 4", "10<Return"] ("Array")) -> ("Selected ID"=w351:i32)  [unwired: 6 in, 1 out]
        n196 = case shown="0, Default" w351 {
          selector: w351 -> [w354 _]
          tunnel: [u32 6 ("Selected ID") 0] -> w350
          frame 0, Default {
            n197 = local write "Sensor Port"(w354) -> ()
          }
          frame 10 {
          }
        }
      }
      frame 5 {
        # "NXT Sensor - MUX"
        n198 = call "DisplayMenu.vi"("Menu Message"="--Select Sensor\nMultiplexer Port--", "2-Digit ID+Character+Message"=string[] [" 0XNo Multiplexer", " 11MUX Port 1", " 22MUX Port 2", " 33MUX Port 3", " 44MUX Port 4", "10<Return"] ("Array")) -> ("Selected ID"=w358:i32)  [unwired: 6 in, 1 out]
        n199 = case shown="10" w358 {
          selector: w358 -> [w361 _]
          tunnel: [u32 9 ("Selected ID") 3] -> w357
          frame 0, Default {
            n200 = local write "MUX Port"(w361) -> ()
          }
          frame 10 {
          }
        }
      }
      frame 6 {
        # "Tetrix Chain Position"
        n201 = local read "Type"() -> (w365:T4)
        n202 = call "DisplayMenu.vi"("Menu Message"="--Select Ctrlr\nChain Position--", "2-Digit ID+Character+Message"=string[] [" 11First Controller", " 22Second Controller", " 33Third Controller", " 44Fourth Controller", "10<Return"] ("Array")) -> ("Selected ID"=w367:i32)  [unwired: 6 in, 1 out]
        n203 = case shown="Default" w365 {
          tunnel: [7 8] -> w364
          frame Default {
          }
          frame "Tetrix Servo" {
          }
        }
        n204 = case shown="0, Default" w367 {
          selector: w367 -> [w372 _]
          tunnel: [w371 4] -> w366
          tunnel: w364 -> [w371 _]
          frame 0, Default {
            n205 = local write "Chain Position"(w372) -> ()
          }
          frame 10 {
          }
        }
      }
      frame 7 {
        # "Tetrix - DC Controller Pos"
        n206 = call "DisplayMenu.vi"("Menu Message"="--Select DC Motor--", "2-Digit ID+Character+Message"=string[] [" 11Motor 1", " 22Motor 2", "10<Return"] ("Array")) -> ("Selected ID"=w376:i32)  [unwired: 6 in, 1 out]
        n207 = case shown="0, Default" w376 {
          selector: w376 -> [w379 _]
          tunnel: [1 6] -> w375
          frame 0, Default {
            n208 = local write "Controller Slot"(w379) -> ()
          }
          frame 10 {
          }
        }
      }
      frame 8 {
        # "Tetrix - Servo Motor Controller Pos"
        n209 = call "DisplayMenu.vi"("Menu Message"="--Select Servo--", "2-Digit ID+Character+Message"=string[] [" 11Servo 1", " 22Servo 2", " 33Servo 3", " 44Servo 4", " 55Servo 5", " 66Servo 6", "10<Return"] ("Array")) -> ("Selected ID"=w383:i32)  [unwired: 6 in, 1 out]
        n210 = case shown="10" w383 {
          selector: w383 -> [w386 _]
          tunnel: [1 6] -> w382
          frame 0, Default {
            n211 = local write "Controller Slot"(w386) -> ()
          }
          frame 10 {
          }
        }
      }
      frame 9 {
        # "NXT Sensor - type"
        n212 = call "DisplayMenu.vi"("Menu Message"="--Select Type--", "2-Digit ID+Character+Message"=string[] [" 0LLight Sensor\nOn", " 1LLight Sensor\nOff", " 2TTouch Sensor", " 3SSound Sensor", " 4UUltrasonic\nSensor", " 5AAccelerometer\nSensor", " 6CCompass Sensor", " 7EEOPD Sensor", " 8FForce Sensor", " 9GGyroscopic\nSensor", "10IIR Seeker v1", "11IIR Seeker v2", "99<Return"] ("Array")) -> ("Selected ID"=w390:i32)  [unwired: 6 in, 1 out]
        n213 = case shown="99" w390 {
          selector: w390 -> [w393 _]
          tunnel: [u32 1 ("Selected ID") 5] -> w389
          frame 0, Default {
            n214 = local write "Sensor Type"(w393) -> ()
          }
          frame 99 {
          }
        }
      }
    }
    n215 = Equal?(x=u32 10000 ("y"), y=w7) -> (x = y?=w6:bool)
    "exit?" <- w6
  }
  n216 = while {
    tunnel: w1 -> [_]
    stop <- w395 stop-if-true
    w401 = T8 3 items=["Enter button"=3, "Left button"=2, "Right button"=1] ("Button (Enter button)")
    w402 = T8 1 items=["Enter button"=3, "Left button"=2, "Right button"=1] ("Button (Enter button)")
    w405 = T8 2 items=["Enter button"=3, "Left button"=2, "Right button"=1] ("Button (Enter button)")
    n217 = call <vilib>:"readNXTButton.vi"("Button (Enter button)"=w405) -> ("Yes/No"=→"Left":bool, "NXT"=w398:T1)  [unwired: 2 in]
    n218 = call <vilib>:"readNXTButton.vi"("Button (Enter button)"=w402, "NXT"=w398) -> ("Yes/No"=→"Right":bool, "NXT"=w397:T1)  [unwired: 1 in]
    n219 = call <vilib>:"readNXTButton.vi"("Button (Enter button)"=w401, "NXT"=w397) -> ("Yes/No"=→"Enter":bool, "NXT"=w396:T1)  [unwired: 1 in]
    n220 = call-poly <vilib>:"PolyWait.vi"("Time (100 msec)"=u32 20, "NXT"=w396) -> ()  [unwired: 2 in, 1 out]
    n221 = local read "exit?"() -> (w395:bool)
  }
  "NXT" <- "NXT"
